vi "Date intrare pentru predictia bolilor de inima.vi"() -> ()   [LabVIEW 2024]
panel:
  out "appended array":dbl[][](array[numeric])
  in  "ritm cardiac minim":dbl
  in  "ritm cardiac maxim":dbl
  in  "rezultatul minim ecg":dbl
  in  "rezultatul maxim ecg":dbl
  in  "nivelul minim de colesterol":dbl
  in  "nivelul maxim de colesterol":dbl
  in  "tensiune arteriala de repaus minima":dbl
  in  "tensiune arteriala de repaus maxima":dbl
  in  "varsta minima":dbl
  in  "varsta maxima":dbl
  in  "val esantion":i32
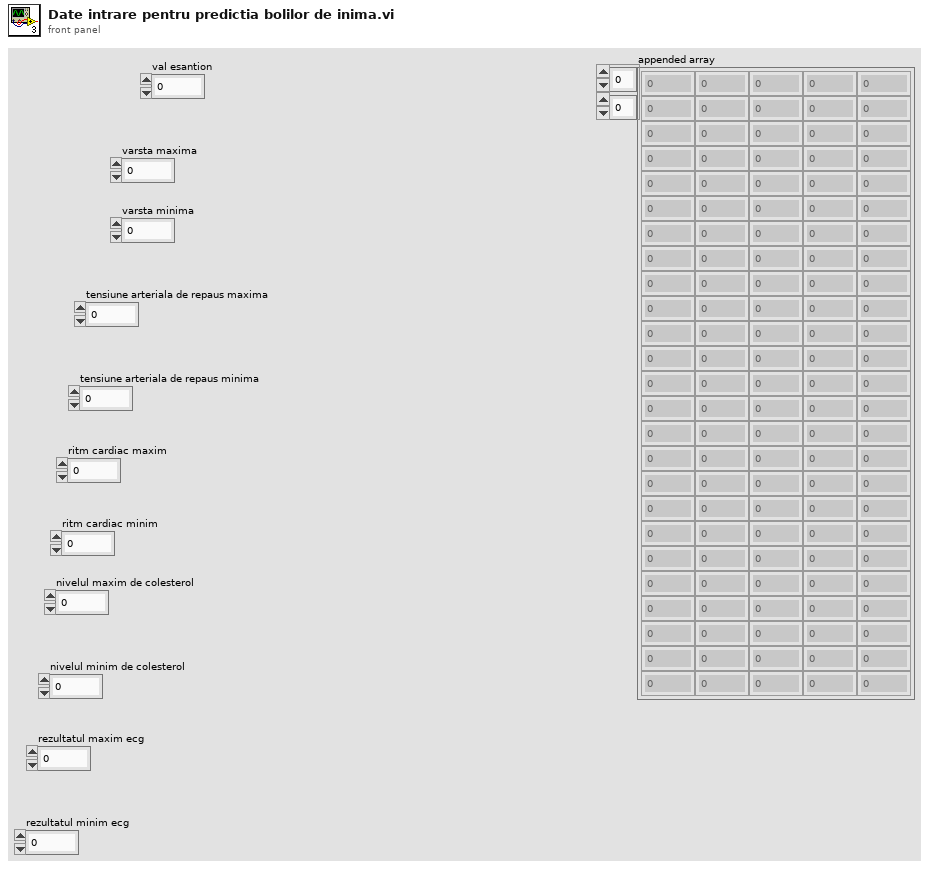
[diagram p1: front panel]
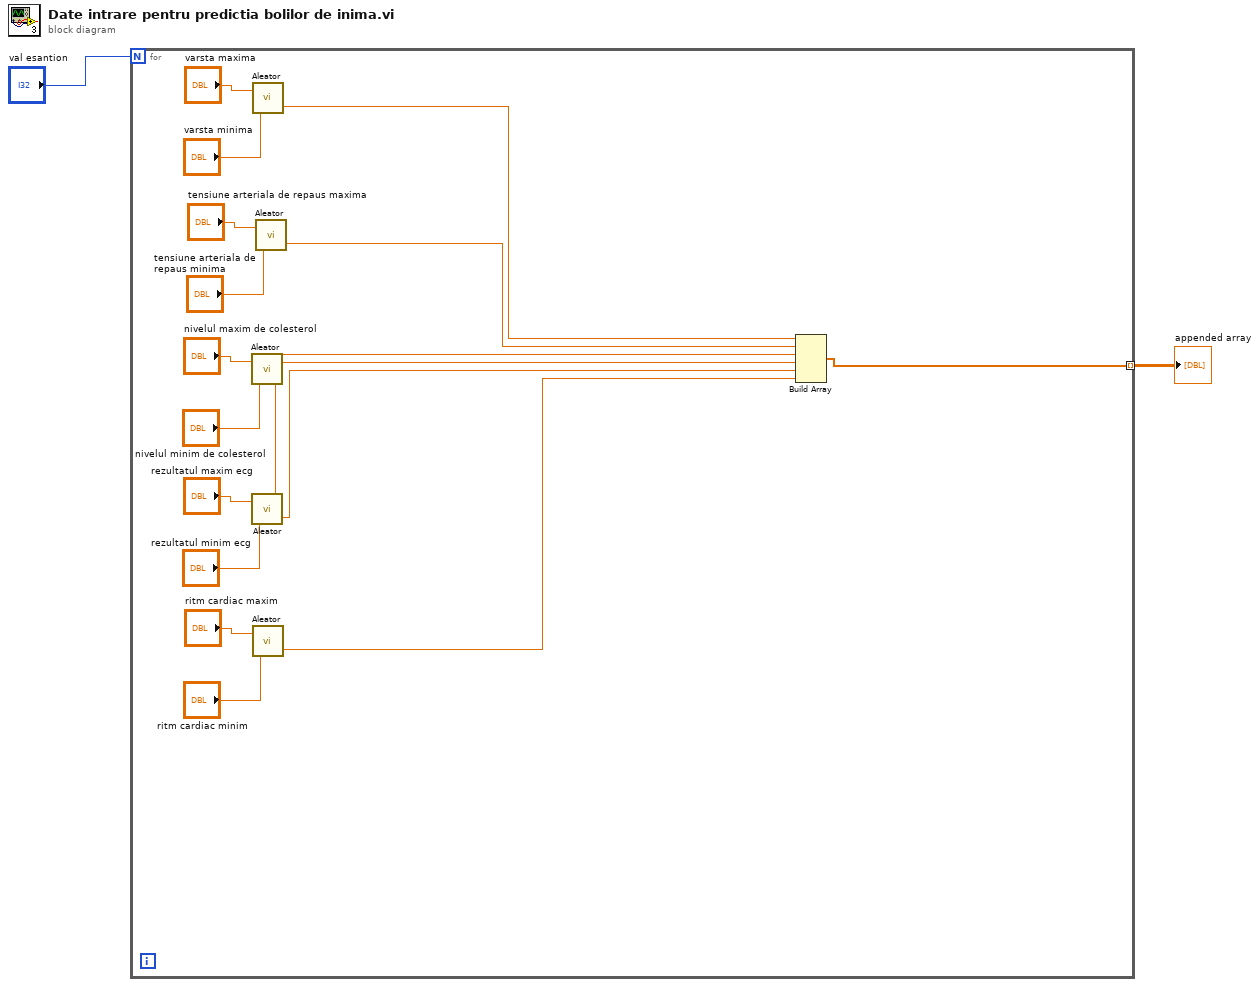
[diagram p0: block diagram]
diagram:
  n1 = for {
    N: "val esantion" -> [_]
    tunnel: [w3] -> w1 mode=indexing
    n2 = call "Aleator.vi"("minim"="nivelul minim de colesterol", "maxim"="nivelul maxim de colesterol") -> ("x val aleatoare"=w6:dbl)  [unwired: 1 in]
    n3 = call "Aleator.vi"("minim"="rezultatul minim ecg", "maxim"="rezultatul maxim ecg") -> ("x val aleatoare"=w5:dbl)  [unwired: 1 in]
    n4 = call "Aleator.vi"("minim"="varsta minima", "maxim"="varsta maxima") -> ("x val aleatoare"=w8:dbl)  [unwired: 1 in]
    n5 = call "Aleator.vi"("minim"="ritm cardiac minim", "maxim"="ritm cardiac maxim") -> ("x val aleatoare"=w4:dbl)  [unwired: 1 in]
    n6 = call "Aleator.vi"("minim"="tensiune arteriala de repaus minima", "maxim"="tensiune arteriala de repaus maxima") -> ("x val aleatoare"=w7:dbl)  [unwired: 1 in]
    n7 = Build Array(w8, w7, w6, w5, w5, w4) -> (w3:dbl[])
  }
  "appended array" <- w1
